vi "Configure Frequency.vi"   [LabVIEW 2018, in "Agilent MXA Series.lvlib"]
doc: "Configures the frequency range for the spectrum analyzer."
uses:
  Agilent MXA Series.lvlib
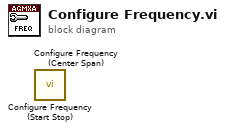
[diagram p0: block diagram]
diagram:
  n1 = call "Configure Frequency (Start Stop).vi"() -> ()  [unwired: 10 in, 2 out]
  n2 = call "Configure Frequency (Center Span).vi"() -> ()  [unwired: 10 in, 2 out]
